vi "Mod3.vi"() -> ()   [LabVIEW 2014]
doc: "\"Discrete LED demo.vi\" -- Demonstrate a discrete LED connected to a digital output.\n\nInstructions:\n\n-- Click the 'enable blinker' button to toggle between blinking mode\nand static mode.\n-- In static mode, click the 'digital level' button to set the state of the\ndigital output.\n-- The 'digital output state' LED indicator shows the state of the\ndigital output (on = high, off = low)."
uses:
  <vilib>/myRIO/Common/Instrument Driver Framework/myRIO v1.0/UART/vis/myRIO v1.0 Close UART.vi
  <vilib>/Utility/error.llb/Error Cluster From Error Code.vi
  <vilib>/myRIO/Common/Instrument Driver Framework/myRIO v1.0/DIO/vis/myRIO v1.0 Write DIO.vi
  <vilib>/myRIO/Common/Instrument Driver Framework/Utilities/vis/FPGA Ref Manager.vi
  <vilib>/myRIO/Common/Instrument Driver Framework/myRIO v1.0/myRIO v1.0 Reset FPGA.vi
  <vilib>/myRIO/Common/Instrument Driver Framework/myRIO v1.0/IRQ/vis/myRIO v1.0 IRQ Info FGV.vi
  <vilib>/myRIO/Common/Instrument Driver Framework/myRIO v1.0/IRQ/vis/myRIO v1.0 Timer IRQ Info FGV.vi
  <vilib>/myRIO/Common/Instrument Driver Framework/myRIO v1.0/IRQ/vis/myRIO v1.0 ISR Agent.vi
  <vilib>/myRIO/Instrument Drivers/Utilities/Utilities.lvlib
  <vilib>/myRIO/Instrument Drivers/Onboard IO/DIO/DIO.lvlib
panel:
  in  "Left/Right":bool
  in  "Control Speed":dbl
  out "error out":errorcluster
  in  "error in (no error)":errorcluster
  in  "[ESC]":bool
  # "7-Segment LED demo"
  # "( The lower the number,\nthe faster it goes"
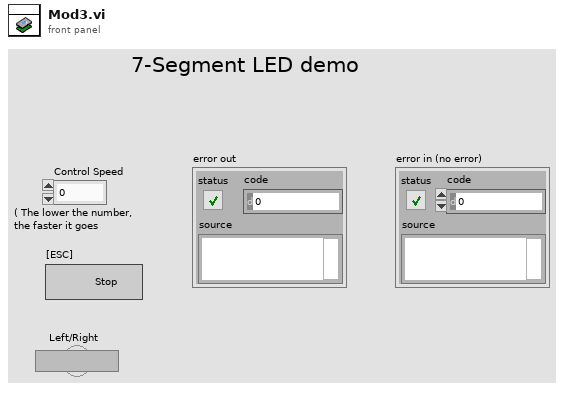
[diagram p1: front panel]
types:
  T1 = typedef "DIO.lvlib/DIO Reference.ctl" = cluster{"myRIO Reference":T2, "DIO Channels List":T6}
  T2 = typedef "myRIO Generic Hardware Reference.ctl" = cluster{"myRIO Model":T3, "myRIO Hardware Reference":T4}
  T3 = typedef "Hardware Version Enum.ctl" = enum16{"Unknown", "myRIO-1900", "myRIO-1950"}
  T4 = typedef "myRIO v1.0 Reference.ctl" = cluster{"Generic FPGA Reference":T5, "Allow multiple opens":bool}
  T5 = typedef "Generic FPGA Reference.ctl" = refnum<k20>
  T6 = typedef "DIO Channels List.ctl" = T7[]
  T7 = typedef "DIO Channels Enum.ctl" = enum16{"Not Connected", "C/DIO0", "C/DIO1", "C/DIO2", "C/DIO3", "C/DIO4", "C/DIO5", "C/DIO6", "C/DIO7", "A/DIO0", "A/DIO1", "A/DIO2", "A/DIO3", "A/DIO4", "A/DIO5", "A/DIO6", "A/DIO7", "A/DIO8", "A/DIO9", "A/DIO10", "A/DIO11", "A/DIO12", "A/DIO13", "A/DIO14", "A/DIO15", "B/DIO0", "B/DIO1", "B/DIO2", "B/DIO3", "B/DIO4", "B/DIO5", "B/DIO6", "B/DIO7", "B/DIO8", "B/DIO9", "B/DIO10", "B/DIO11", "B/DIO12", "B/DIO13", "B/DIO14", "B/DIO15", "LED0", "LED1", "LED2", "LED3", "Button0"}
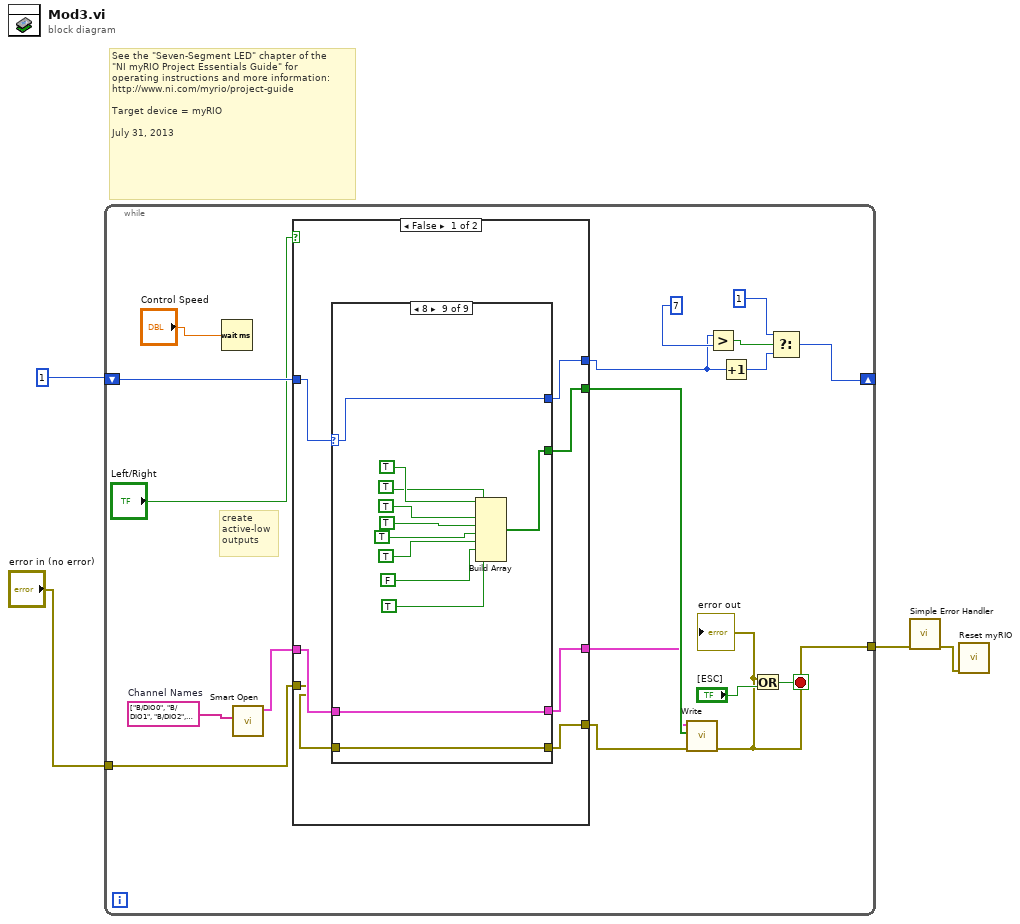
[diagram p0: block diagram]
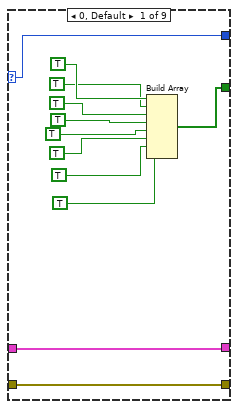
[diagram p2: hidden frame]
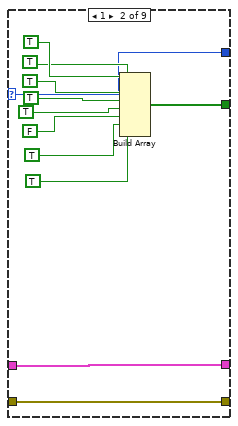
[diagram p3: hidden frame]
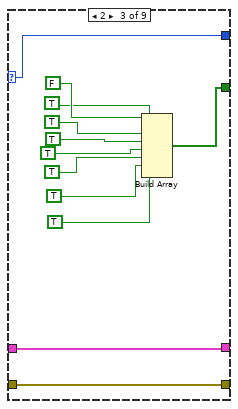
[diagram p4: hidden frame]
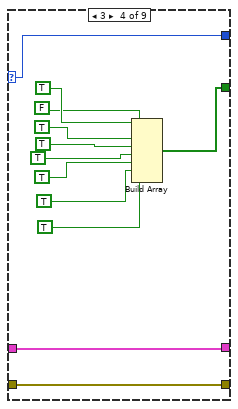
[diagram p5: hidden frame]
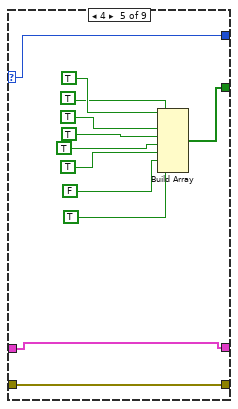
[diagram p6: hidden frame]
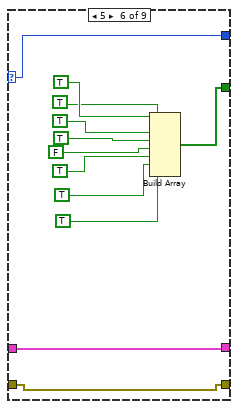
[diagram p7: hidden frame]
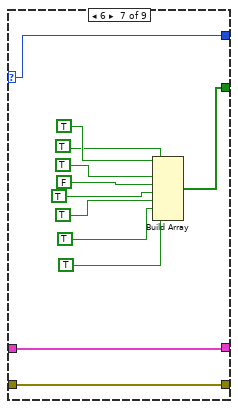
[diagram p8: hidden frame]
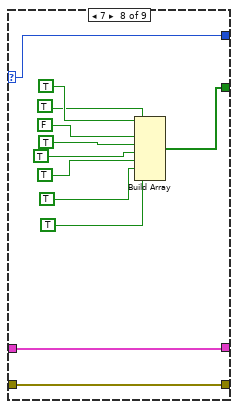
[diagram p9: hidden frame]
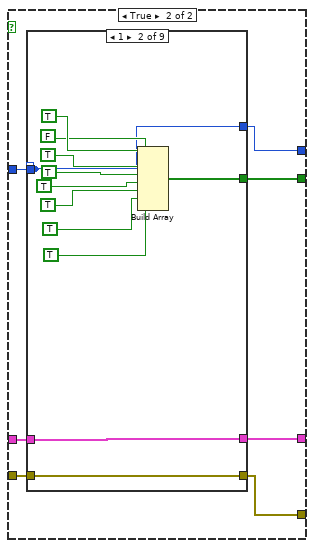
[diagram p10: hidden frame]
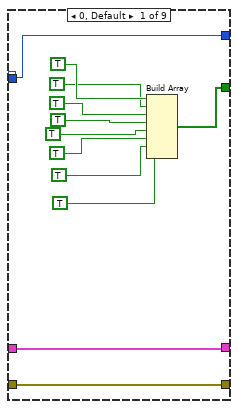
[diagram p11: hidden frame]
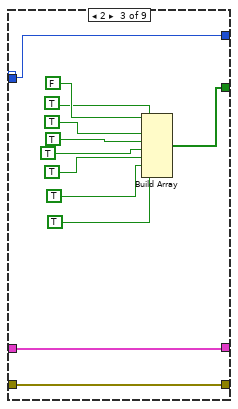
[diagram p12: hidden frame]
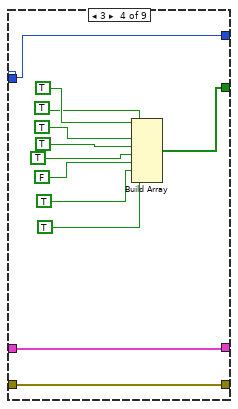
[diagram p13: hidden frame]
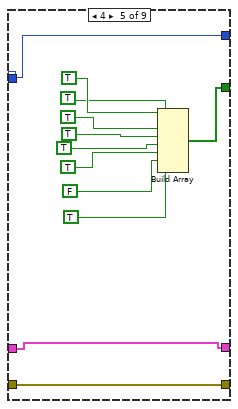
[diagram p14: hidden frame]
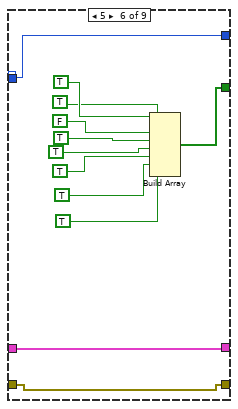
[diagram p15: hidden frame]
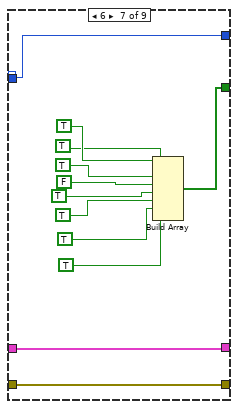
[diagram p16: hidden frame]
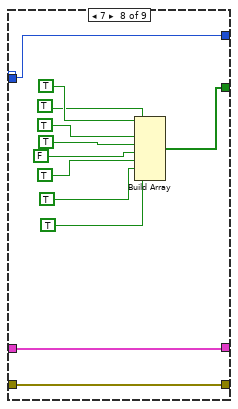
[diagram p17: hidden frame]
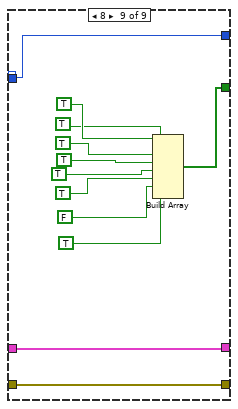
[diagram p18: hidden frame]
diagram:
  # "See the \"Seven-Segment LED\" chapter of the\n\"NI myRIO Project Essentials Guide\" for\noperating instructions and more information: \nhttp://www.ni.com/myrio/project-guide\n\nTarget device = myRIO\n\nJuly 31, 2013"
  n1 = while {
    tunnel: [w9] -> w3
    tunnel: "error in (no error)" -> [w12]
    shift-right: [w15] -> _
    shift-left: 1 -> [w11]
    stop <- w22 stop-if-true
    w20 = tag[] ["B/DIO0", "B/DIO1", "B/DIO2", "B/DIO3", "B/DIO4", "B/DIO5", "B/DIO6", "B/DIO7"]  # Channel Names
    # "create\nactive-low\noutputs"
    n2 = Wait (ms)(milliseconds to wait="Control Speed") -> ()  [unwired: 1 out]
    n3 = call <vilib>:"Smart Open.vi"("Channel Names"=w20) -> ("DIO Ref Out"=w13:T1)  [unwired: 9 in, 1 out]
    n4 = case shown="False" "Left/Right" {
      tunnel: w13 -> [w26 w144]
      tunnel: w12 -> [w23 w141]
      tunnel: [w29 w142] -> w10
      tunnel: w11 -> [w27 w143]
      tunnel: [w24 w140] -> w8
      tunnel: [w25 w139] -> w6
      tunnel: [w28 w138] -> w7
      frame False {
        n5 = case shown="8" w27 {
          selector: w27 -> [w30 w42 w54 w66 w78 w90 w102 w114 w126]
          tunnel: [w40 w53 w56 w68 w80 w92 w104 w117 w129] -> w25
          tunnel: w26 -> [w40 w53 w56 w68 w80 w92 w104 w117 w129]
          tunnel: w23 -> [w41 w52 w55 w67 w79 w91 w105 w116 w128]
          tunnel: [w41 w52 w55 w67 w79 w91 w105 w116 w128] -> w24
          tunnel: [w32 w43 w57 w69 w81 w93 w103 w115 w127] -> w28
          tunnel: [w30 w42 w54 w66 w78 w90 w102 w114 w126] -> w29
          frame 0, Default {
            n6 = Build Array(TRUE, TRUE, TRUE, TRUE, TRUE, TRUE, TRUE, TRUE) -> (w32:bool[])
          }
          frame 1 {
            n7 = Build Array(TRUE, TRUE, TRUE, TRUE, TRUE, FALSE, TRUE, TRUE) -> (w43:bool[])
          }
          frame 2 {
            n8 = Build Array(FALSE, TRUE, TRUE, TRUE, TRUE, TRUE, TRUE, TRUE) -> (w57:bool[])
          }
          frame 3 {
            n9 = Build Array(TRUE, FALSE, TRUE, TRUE, TRUE, TRUE, TRUE, TRUE) -> (w69:bool[])
          }
          frame 4 {
            n10 = Build Array(TRUE, TRUE, TRUE, TRUE, TRUE, TRUE, FALSE, TRUE) -> (w81:bool[])
          }
          frame 5 {
            n11 = Build Array(TRUE, TRUE, TRUE, TRUE, FALSE, TRUE, TRUE, TRUE) -> (w93:bool[])
          }
          frame 6 {
            n12 = Build Array(TRUE, TRUE, TRUE, FALSE, TRUE, TRUE, TRUE, TRUE) -> (w103:bool[])
          }
          frame 7 {
            n13 = Build Array(TRUE, TRUE, FALSE, TRUE, TRUE, TRUE, TRUE, TRUE) -> (w115:bool[])
          }
          frame 8 {
            n14 = Build Array(TRUE, TRUE, TRUE, TRUE, TRUE, TRUE, FALSE, TRUE) -> (w127:bool[])
          }
        }
      }
      frame True {
        n15 = case shown="1" w143 {
          selector: w143 -> [w145 w157 w169 w181 w193 w205 w217 w229 w241]
          tunnel: [w155 w168 w171 w183 w195 w207 w219 w232 w244] -> w139
          tunnel: w144 -> [w155 w168 w171 w183 w195 w207 w219 w232 w244]
          tunnel: w141 -> [w156 w167 w170 w182 w194 w206 w220 w231 w243]
          tunnel: [w156 w167 w170 w182 w194 w206 w220 w231 w243] -> w140
          tunnel: [w147 w158 w172 w184 w196 w208 w218 w230 w242] -> w138
          tunnel: [w145 w157 w169 w181 w193 w205 w217 w229 w241] -> w142
          tunnel: w143 -> [_ _ _ _ _ _ _ _ _]
          frame 0, Default {
            n16 = Build Array(TRUE, TRUE, TRUE, TRUE, TRUE, TRUE, TRUE, TRUE) -> (w147:bool[])
          }
          frame 1 {
            n17 = Build Array(TRUE, FALSE, TRUE, TRUE, TRUE, TRUE, TRUE, TRUE) -> (w158:bool[])
          }
          frame 2 {
            n18 = Build Array(FALSE, TRUE, TRUE, TRUE, TRUE, TRUE, TRUE, TRUE) -> (w172:bool[])
          }
          frame 3 {
            n19 = Build Array(TRUE, TRUE, TRUE, TRUE, TRUE, FALSE, TRUE, TRUE) -> (w184:bool[])
          }
          frame 4 {
            n20 = Build Array(TRUE, TRUE, TRUE, TRUE, TRUE, TRUE, FALSE, TRUE) -> (w196:bool[])
          }
          frame 5 {
            n21 = Build Array(TRUE, TRUE, FALSE, TRUE, TRUE, TRUE, TRUE, TRUE) -> (w208:bool[])
          }
          frame 6 {
            n22 = Build Array(TRUE, TRUE, TRUE, FALSE, TRUE, TRUE, TRUE, TRUE) -> (w218:bool[])
          }
          frame 7 {
            n23 = Build Array(TRUE, TRUE, TRUE, TRUE, FALSE, TRUE, TRUE, TRUE) -> (w230:bool[])
          }
          frame 8 {
            n24 = Build Array(TRUE, TRUE, TRUE, TRUE, TRUE, TRUE, FALSE, TRUE) -> (w242:bool[])
          }
        }
      }
    }
    n25 = call <vilib>:"Write.vi"("error in (no error)"=w8, "Values"=w7, "DIO Ref In"=w6) -> ("error out"=w9:errorcluster)  [unwired: 6 in, 1 out]
    "error out" <- w9
    n26 = Greater?(x=w10, y=7) -> (0:w18:bool)
    n27 = Increment(x=w10) -> (x+1=w14:i32)
    n28 = Or(x=w9, y="[ESC]") -> (x .or. y?=w22:bool)
    n29 = Select(t=1, s=w18, f=w14) -> (s? t:f=w15:i32)
  }
  n30 = call <vilib>:"Simple Error Handler.vi"("error in (no error)"=w3) -> ("error out"=w4:errorcluster)  [unwired: 4 in, 4 out]
  n31 = call <vilib>:"Reset myRIO.vi"("error in (no error)"=w4) -> ()  [unwired: 10 in, 1 out]
